vi "AIT 1553 - Conditionally Serialize.vi"(8 "error in (no error)":errorcluster, 11 "Device Item Ref in":T1 format="%.0x") -> (0 "error out":errorcluster)   [LabVIEW 2013, in "AIT 1553 Custom Device.lvlib"]
uses:
  AIT 1553 Custom Device.lvlib
  <vilib>/NI Veristand/Custom Device API/Custom Device Item Ref.ctl
  Controls and Global/Global.vi
  <vilib>/NI Veristand/Custom Device API/Get Item Property (Path).vi
  <vilib>/NI Veristand/Custom Device API/NI VeriStand - Add Custom Device Dependencies.vi
  <vilib>/NI Veristand/Custom Device API/NI VeriStand - Reset Custom Device Dependencies.vi
  <vilib>/NI Veristand/Custom Device API/Custom Device API.lvlib
  <vilib>/NI Veristand/Custom Device Tools/Custom Device Utility Library/Custom Device Utility Library.lvlib
  <vilib>/NI Veristand/Custom Device Tools/Custom Device Utility Library/NI VeriStand - Search for Item by GUID.vi
  <vilib>/NI Veristand/Custom Device Tools/Custom Device Utility Library/Search Direction.ctl
panel:
  out "Converted File":path
  out "Value":path
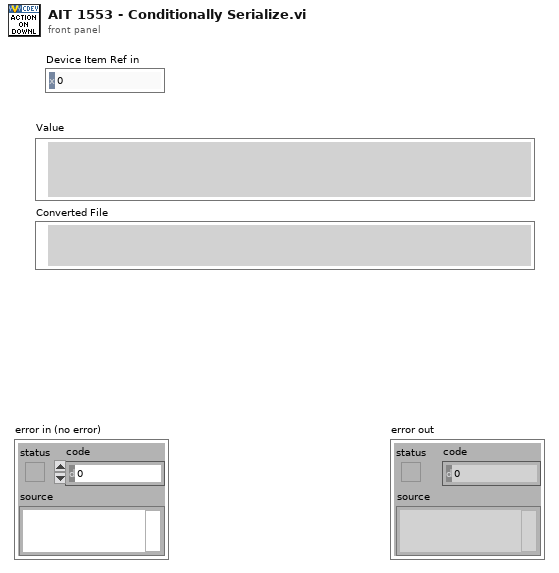
[diagram p1: front panel]
types:
  T1 = typedef "Custom Device API.lvlib/Custom Device Item Ref.ctl" = u64
  T2 = typedef "Custom Device Utility Library.lvlib/Search Direction.ctl" = enum16{"Down", "Up"}
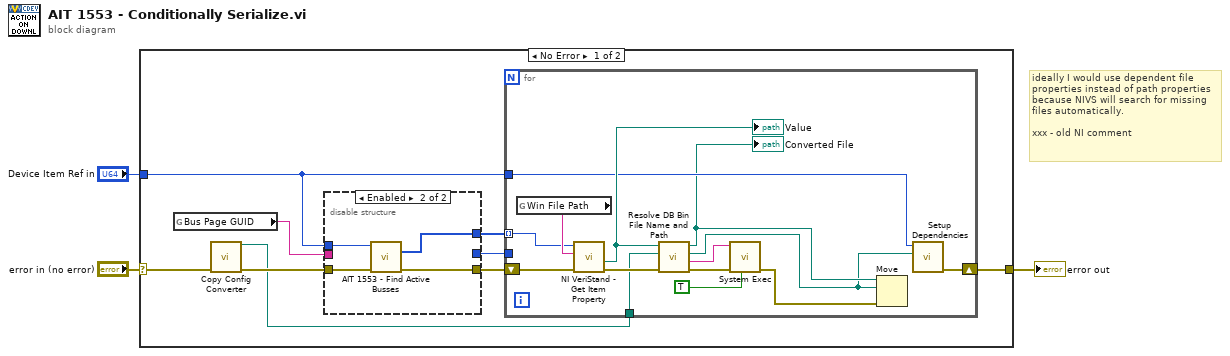
[diagram p0: block diagram]
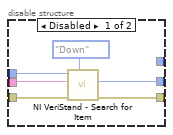
[diagram p2: hidden frame]
diagram:
  # "ideally I would use dependent file properties instead of path properties because NIVS will search for missing files automatically.\n\nxxx - old NI comment"
  n1 = case shown="No Error" "error in (no error)" {
    selector: "error in (no error)" -> [w11 w37]
    tunnel: [w12 w37] -> w2
    tunnel: "Device Item Ref in" -> [w7 _]
    frame No Error {
      n2 = global read "Global.vi" "Bus Page GUID"() -> (w5:string)
      n3 = call "Copy Config Converter.vi"("error in (no error)"=w11) -> ("original path to converter"=w4:path, "error out"=w10:errorcluster)  [unwired: 13 in]
      n4 = disable-structure shown="Enabled" {
        disable-tunnel: w5 -> [w32 _]
        disable-tunnel: w10 -> [w30 w36]
        disable-tunnel: [w29 w35] -> w9
        disable-tunnel: w7 -> [w28 w33]
        disable-tunnel: [w27 _] -> w8
        disable-tunnel: [_ w34] -> w6
        frame Disabled {
          n5 = call-poly <vilib>:"NI VeriStand - Search for Item.vi"("Direction (Down)"=Search_Direction."Down", "error in"=w30, "Item GUID"=w32, "Section Ref in"=w28) -> ("error out"=w29:errorcluster, "Item Ref"=w27:T1)  [unwired: 4 in, 2 out]
        }
        frame Enabled {
          n6 = call "AIT 1553 - Find Active Busses.vi"("Device Item Ref in"=w33, "error in (no error)"=w36) -> ("Child Refs - 1553 Busses"=w34:T1[], "error out"=w35:errorcluster)  [unwired: 11 in, 1 out]
        }
      }
      n7 = for {
        tunnel: w8 -> [_]
        tunnel: w7 -> [w19]
        tunnel: w6 -> [w18] mode=indexing
        shift-right: [w26] -> w12
        shift-left: w9 -> [w25]
        tunnel: w4 -> [w17]
        n8 = global read "Global.vi" "Win File Path"() -> (w24:string)
        n9 = call-poly <vilib>:"NI VeriStand - Get Item Property.vi"("error in (no error)"=w25, "Property Name"=w24, "Item Ref in"=w18) -> ("error out"=w22:errorcluster, "Value"=w20:path)  [unwired: 5 in, 2 out]
        "Value" <- w20
        n10 = call "Resolve DB Bin File Name and Path.vi"("error in"=w22, "Path to Tools"=w17, "DB XML File"=w20) -> ("error out"=w21:errorcluster, "SysExec"=w16:string, "Converted File Destination"=w13:path, "Converted File Source"=w14:path)  [unwired: 5 in]
        "Converted File" <- w14
        n11 = call <vilib>:"System Exec.vi"("run minimized? (F)"=TRUE, "error in (no error)"=w21, "command line"=w16) -> ("error out"=w15:errorcluster)  [unwired: 5 in, 3 out]
        n12 = Move(source path=w14, error in=w15, 10:w13) -> ()  [unwired: 2 in, 3 out]
        n13 = call "Setup Dependencies.vi"("Windows Bin File"=w13, "Item Ref in"=w19) -> ("error out"=w26:errorcluster)  [unwired: 9 in]
      }
    }
    frame Error {
    }
  }
  "error out" <- w2
